vi "PERFORMANCE FUNCTIONS.vi"(0 "Source Name":string="Source Name", 11 "Error In Cluster":T1={"Unhandled Error"=FALSE, "Error"={"status"=FALSE, "code"=0, "source"=""}, "Message Type"=enum."Code", "Number of Values"=0, "Msg Value Type"=[], "Msg Ints"=[], "Msg Real Values"=[], "Msg String Values"=[], "Severity (Emergency)"=enum."Emergency"} {"Msg Real Values" format="%.2f"}) -> (15 "Error Out Cluster":T2={"Unhandled Error"=FALSE, "Error"={"status"=FALSE, "code"=0, "source"=""}, "Message Type"=enum."Code", "Number of Values"=0, "Msg Value Type"=[], "Msg Ints"=[], "Msg Real Values"=[], "Msg String Values"=[], "Severity (Emergency)"=enum."Emergency"} {"Msg Real Values" format="%.2f"})   [LabVIEW 2013, in "Customer.TestSLATE.Mnemonic.lvlib"]
doc: "XXX PERFORMANCE FUNCTIONS.vi monitors the current command set active for the data manager running under the DTMGR EXEC and performs each command as it is received. Valid commands are INIT (Initialize system), ACQ (Data Acquisition), DIAG (Diagnostics), STOP (No command active, but data collection will be performed), CAL\n(Calibration), and RELOAD DB (Collect new required configuration database files)."
uses:
  Customer.TestSLATE.Mnemonic.lvlib
  <vilib>/Test SLATE/CONTROLS/Error Out Cluster.ctl
  <vilib>/Test SLATE/CONTROLS/Error In Cluster.ctl
  <vilib>/Test SLATE/Test SLATE.lvlib
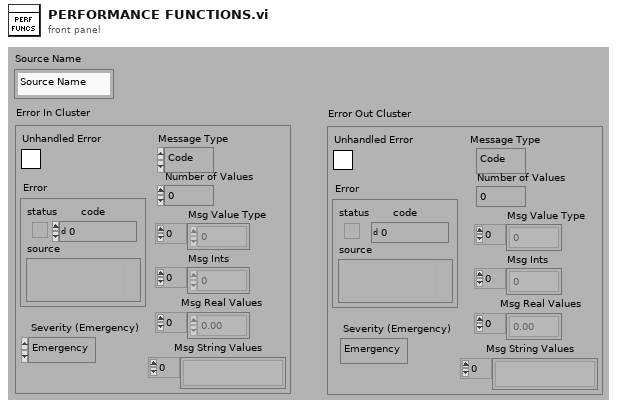
[diagram p1: front panel]
types:
  T1 = typedef "Test SLATE.lvlib/Error In Cluster.ctl" = cluster{"Unhandled Error":bool, "Error":errorcluster, "Message Type":enum8{"Code", "Text"}, "Number of Values":i8, "Msg Value Type":i32[], "Msg Ints":i32[], "Msg Real Values":sgl[], "Msg String Values":string[], "Severity (Emergency)":enum32{"Information", "Warning", "Emergency"}}
  T2 = typedef "Test SLATE.lvlib/Error Out Cluster.ctl" = cluster{"Unhandled Error":bool, "Error":errorcluster, "Message Type":enum8{"Code", "Text"}, "Number of Values":i8, "Msg Value Type":i32[], "Msg Ints":i32[], "Msg Real Values":sgl[], "Msg String Values":string[], "Severity (Emergency)":enum32{"Information", "Warning", "Emergency"}}
  T3 = typedef "Test SLATE.lvlib/Tag Information.ctl" = refnum<class "TS_Tag.lvclass">
  T4 = typedef "Test SLATE.lvlib/CALIBRATION TYPE EXEC.ctl" = enum16{"End to End", "Special 1", "Special 2", "Special 3", "Waiting for Type", "Special 4", "Special 5"}
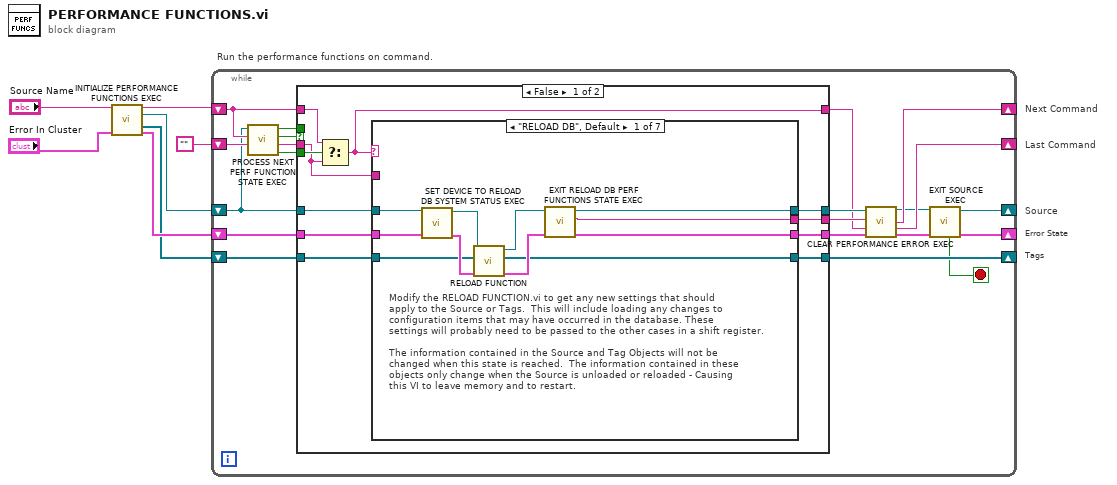
[diagram p0: block diagram]
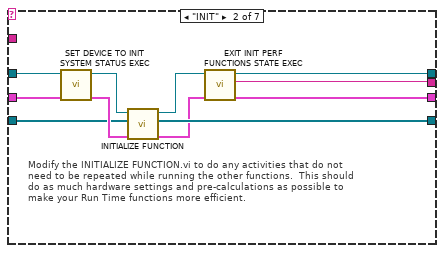
[diagram p2: hidden frame]
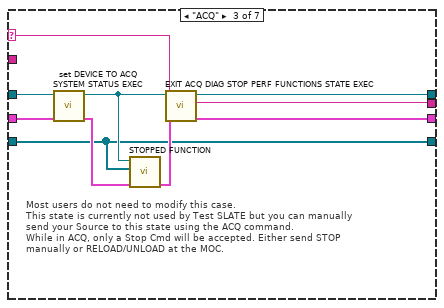
[diagram p3: hidden frame]
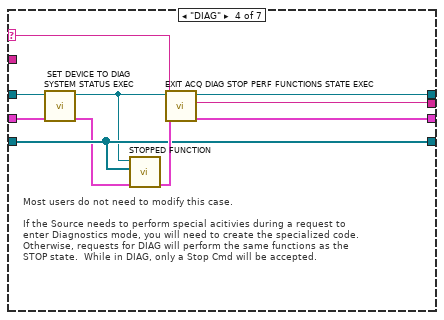
[diagram p4: hidden frame]
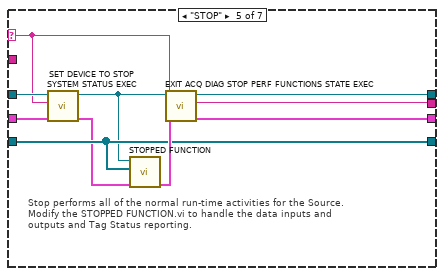
[diagram p5: hidden frame]
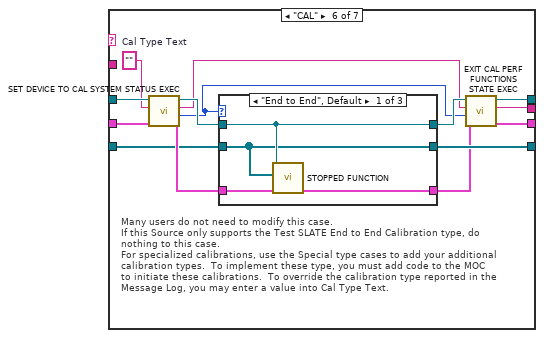
[diagram p6: hidden frame]
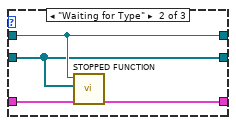
[diagram p7: hidden frame]
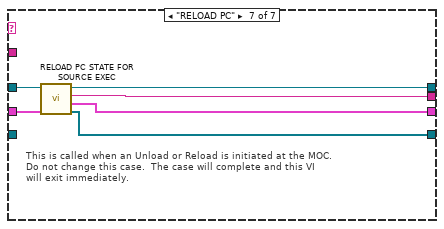
[diagram p9: hidden frame]
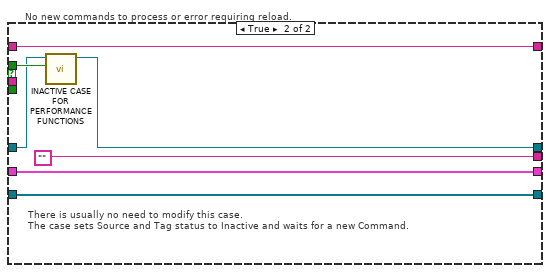
[diagram p10: hidden frame]
diagram:
  # "Tags"
  # "Error State"
  # "Source"
  # "Last Command"
  # "Next Command"
  # "Run the performance functions on command."
  n1 = call <vilib>:"INITIALIZE PERFORMANCE FUNCTIONS EXEC.vi"("Source Name"="Source Name", "Error In Cluster"="Error In Cluster") -> ("Init Command"=w5:string, "Source"=w2:refnum<class "Source.lvclass">, "Tags"=w1:T3[], "Error Out Cluster"=w7:T1)  [unwired: 9 in, 1 out]
  n2 = while {
    shift-left: w5 -> [w19]
    shift-right: [w16] -> _
    shift-left: "" -> [w28]
    shift-right: [w13] -> _
    shift-left: w7 -> [w27]
    shift-right: [w9] -> _
    shift-right: [w21] -> _
    shift-left: w1 -> [w20]
    shift-right: [w11] -> _
    shift-left: w2 -> [w18]
    stop <- w8 stop-if-true
    n3 = call <vilib>:"PROCESS NEXT PERF FUNCTION STATE EXEC.vi"("Last Command"=w28, "Next Command From DTMGR"=w19, "Source"=w18) -> ("Use DTMGR Cmd?"=w26:bool, "Current Command"=w22:string, "Go INACTIVE?"=w25:bool, "MOC sent INACTIVE CMD?"=w23:bool)  [unwired: 5 in]
    n4 = case shown="False" w25 {
      tunnel: [w33 w129] -> w24
      tunnel: w27 -> [w38 w129]
      tunnel: w22 -> [w35 _]
      tunnel: w19 -> [w36 w126]
      tunnel: [w39 w123] -> w15
      tunnel: w26 -> [w37 _]
      tunnel: [w34 w126] -> w14
      tunnel: w23 -> [_ w128]
      tunnel: w18 -> [w32 w124]
      tunnel: [w31 w127] -> w21
      tunnel: w20 -> [w30 w127]
      tunnel: [w29 ""] -> w17
      frame False {
        n5 = Select(t=w36, s=w37, f=w35) -> (s? t:f=w34:string)
        n6 = case shown="\"RELOAD DB\", Default" w34 {
          selector: w34 -> [_ _ w68 w81 w85 _ _]
          tunnel: [w44 w58 w65 w79 w90 w96 w120] -> w33
          tunnel: [w43 w61 w64 w78 w89 w98 w118] -> w39
          tunnel: w38 -> [w50 w59 w71 w75 w86 w105 w121]
          tunnel: w35 -> [_ _ _ _ _ _ _]
          tunnel: w32 -> [w49 w60 w70 w76 w87 w104 w122]
          tunnel: [w45 w55 w63 w77 w88 w100 w119] -> w31
          tunnel: w30 -> [w40 w52 w63 w77 w88 w101 _]
          tunnel: [w41 w51 w62 w72 w82 w95 w117] -> w29
          frame "RELOAD DB", Default {
            # "Modify the RELOAD FUNCTION.vi to get any new settings that should\napply to the Source or Tags.  This will include loading any changes to\nconfiguration items that may have occurred in the database. These \nsettings will probably need to be passed to the other cases in a shift register.\n\nThe information contained in the Source and Tag Objects will not be\nchanged when this state is reached.  The information contained in these\nobjects only change when the Source is unloaded or reloaded - Causing\nthis VI to leave memory and to restart."
            n7 = call <vilib>:"SET DEVICE TO RELOAD DB SYSTEM STATUS EXEC.vi"("Error In Cluster"=w50, "Source"=w49) -> ("Error Out Cluster"=w47:T2, "Source out"=w48:refnum<class "Source.lvclass">)  [unwired: 8 in]
            n8 = call "RELOAD FUNCTION.vi"("Error In Cluster"=w47, "Tags"=w40, "Source"=w48) -> ("Error Out Cluster"=w46:T2, "Tags Out"=w45:T3[], "Source out"=w42:refnum<class "Source.lvclass">)  [unwired: 6 in]
            n9 = call <vilib>:"EXIT RELOAD DB PERF FUNCTIONS STATE EXEC.vi"("Error In Cluster"=w46, "Source"=w42) -> ("Error Out Cluster"=w44:T2, "Next Command"=w41:string, "Source Out"=w43:refnum<class "Source.lvclass">)  [unwired: 7 in]
          }
          frame "INIT" {
            # "Modify the INITIALIZE FUNCTION.vi to do any activities that do not \nneed to be repeated while running the other functions.  This should\ndo as much hardware settings and pre-calculations as possible to\nmake your Run Time functions more efficient."
            n10 = call <vilib>:"SET DEVICE TO INIT SYSTEM STATUS EXEC.vi"("Error In Cluster"=w59, "Source"=w60) -> ("Error Out Cluster"=w54:T1, "Source out"=w57:refnum<class "Source.lvclass">)  [unwired: 6 in]
            n11 = call "INITIALIZE FUNCTION.vi"("Error In Cluster"=w54, "Tags"=w52, "Source"=w57) -> ("Error Out Cluster"=w53:T2, "Tags out"=w55:T3[], "Source out"=w56:refnum<class "Source.lvclass">)  [unwired: 6 in]
            n12 = call <vilib>:"EXIT INIT PERF FUNCTIONS STATE EXEC.vi"("Error In Cluster"=w53, "Source"=w56) -> ("Error Out Cluster"=w58:T1, "Next Command Step"=w51:string, "Source out"=w61:refnum<class "Source.lvclass">)  [unwired: 5 in]
          }
          frame "ACQ" {
            # "Most users do not need to modify this case.\nThis state is currently not used by Test SLATE but you can manually\nsend your Source to this state using the ACQ command.  \nWhile in ACQ, only a Stop Cmd will be accepted. Either send STOP\nmanually or RELOAD/UNLOAD at the MOC."
            n13 = call <vilib>:"set DEVICE TO ACQ SYSTEM STATUS EXEC.vi"("Error In"=w71, "Source"=w70) -> ("Error Out Cluster"=w69:T2, "Source out"=w66:refnum<class "Source.lvclass">)  [unwired: 8 in]
            n14 = call "STOPPED FUNCTION.vi"("Error In Cluster"=w69, "Tags"=w63, "Source"=w66) -> ("Error Out Cluster"=w67:T2)  [unwired: 8 in]
            n15 = call <vilib>:"EXIT ACQ DIAG STOP PERF FUNCTIONS STATE EXEC.vi"("Error In Cluster"=w67, "Command"=w68, "Source"=w66) -> ("Error Out Cluster"=w65:T2, "Next Command"=w62:string, "Source Out"=w64:refnum<class "Source.lvclass">)  [unwired: 6 in]
          }
          frame "DIAG" {
            # "Most users do not need to modify this case.\n\nIf the Source needs to perform special acitivies during a request to\nenter Diagnostics mode, you will need to create the specialized code.\nOtherwise, requests for DIAG will perform the same functions as the \nSTOP state.  While in DIAG, only a Stop Cmd will be accepted."
            n16 = call <vilib>:"SET DEVICE TO DIAG SYSTEM STATUS EXEC.vi"("Error In Cluster"=w75, "Source"=w76) -> ("Error Out Cluster"=w74:T2, "Source out"=w73:refnum<class "Source.lvclass">)  [unwired: 8 in]
            n17 = call "STOPPED FUNCTION.vi"("Error In Cluster"=w74, "Tags"=w77, "Source"=w73) -> ("Error Out Cluster"=w80:T2)  [unwired: 8 in]
            n18 = call <vilib>:"EXIT ACQ DIAG STOP PERF FUNCTIONS STATE EXEC.vi"("Error In Cluster"=w80, "Command"=w81, "Source"=w73) -> ("Error Out Cluster"=w79:T2, "Next Command"=w72:string, "Source Out"=w78:refnum<class "Source.lvclass">)  [unwired: 6 in]
          }
          frame "STOP" {
            # "Stop performs all of the normal run-time activities for the Source.\nModify the STOPPED FUNCTION.vi to handle the data inputs and\noutputs and Tag Status reporting."
            n19 = call <vilib>:"SET DEVICE TO STOP SYSTEM STATUS EXEC.vi"("Error In Cluster"=w86, "MOC Command"=w85, "Source"=w87) -> ("Error Out Cluster"=w83:T2, "Source out"=w84:refnum<class "Source.lvclass">)  [unwired: 6 in]
            n20 = call "STOPPED FUNCTION.vi"("Error In Cluster"=w83, "Tags"=w88, "Source"=w84) -> ("Error Out Cluster"=w91:T2)  [unwired: 8 in]
            n21 = call <vilib>:"EXIT ACQ DIAG STOP PERF FUNCTIONS STATE EXEC.vi"("Error In Cluster"=w91, "Command"=w85, "Source"=w84) -> ("Error Out Cluster"=w90:T2, "Next Command"=w82:string, "Source Out"=w89:refnum<class "Source.lvclass">)  [unwired: 6 in]
          }
          frame "CAL" {
            w92 = ""  # Cal Type Text
            # "Many users do not need to modify this case.\nIf this Source only supports the Test SLATE End to End Calibration type, do\nnothing to this case.\nFor specialized calibrations, use the Special type cases to add your additional\ncalibration types.  To implement these type, you must add code to the MOC\nto initiate these calibrations.  To override the calibration type reported in the\nMessage Log, you may enter a value into Cal Type Text."
            n22 = call <vilib>:"SET DEVICE TO CAL SYSTEM STATUS EXEC.vi"("Error In Cluster"=w105, "Cal Type Text"=w92, "Source"=w104) -> ("Error Out Cluster"=w103:T2, "Calibration Type"=w93:T4, "Cal Type Text Out"=w94:string, "Source out"=w102:refnum<class "Source.lvclass">)  [unwired: 4 in]
            n23 = case shown="\"End to End\", Default" w93 {
              tunnel: w103 -> [w109 w113 w115]
              tunnel: [w108 w112 w115] -> w97
              tunnel: w102 -> [w107 w111 w116]
              tunnel: w101 -> [w106 w110 w114]
              tunnel: [w107 w111 w116] -> w99
              tunnel: [w106 w110 w114] -> w100
              frame "End to End", Default {
                n24 = call "STOPPED FUNCTION.vi"("Error In Cluster"=w109, "Tags"=w106, "Source"=w107) -> ("Error Out Cluster"=w108:T2)  [unwired: 8 in]
              }
              frame "Waiting for Type" {
                # "Put the waiting code here.  \nUsually the same \nas stopped (idle mode)."
                n25 = call "STOPPED FUNCTION.vi"("Error In Cluster"=w113, "Tags"=w110, "Source"=w111) -> ("Error Out Cluster"=w112:T2)  [unwired: 8 in]
              }
              frame "Special 1".."Special 3" {
                # "Add whatever you need for\nthese calibrations.  Use Stop\nAvailable to tell the cmd interface\nif stop commands are available."
              }
            }
            n26 = call <vilib>:"EXIT CAL PERF FUNCTIONS STATE EXEC.vi"("Error In Cluster"=w97, "Calibration Type"=w93, "Cal Type String"=w94, "Source"=w99) -> ("Error Out Cluster"=w96:T2, "Next Command"=w95:string, "Source Out"=w98:refnum<class "Source.lvclass">)  [unwired: 5 in]
          }
          frame "RELOAD PC" {
            # "This is called when an Unload or Reload is initiated at the MOC.\nDo not change this case.  The case will complete and this VI\nwill exit immediately."
            n27 = call <vilib>:"RELOAD PC STATE FOR SOURCE EXEC.vi"("Error In Cluster"=w121, "Source"=w122) -> ("Tags"=w119:T3[], "Error Out Cluster"=w120:T2, "Next Command"=w117:string, "Source Out"=w118:refnum<class "Source.lvclass">)  [unwired: 6 in]
          }
        }
        "Error Out Cluster" <- w33
      }
      frame True {
        # "There is usually no need to modify this case.\nThe case sets Source and Tag status to Inactive and waits for a new Command."
        # "No new commands to process or error requiring reload."
        n28 = call <vilib>:"INACTIVE CASE FOR PERFORMANCE FUNCTIONS.vi"("Stop Status Update Value"=w128, "Source"=w124) -> ("Source Out"=w123:refnum<class "Source.lvclass">)  [unwired: 9 in]
      }
    }
    n29 = call <vilib>:"CLEAR PERFORMANCE ERROR EXEC.vi"("Source"=w15, "Next Command in"=w17, "Last Command in"=w14, "Error In Cluster"=w24) -> ("Source out"=w12:refnum<class "Source.lvclass">, "Next Command Out"=w16:string, "Last Command out"=w13:string, "Error Out Cluster"=w10:T2)  [unwired: 8 in]
    n30 = call <vilib>:"EXIT SOURCE EXEC.vi"("Error In Cluster"=w10, "Source in"=w12) -> ("Error Out Cluster"=w9:T2, "Source out"=w11:refnum<class "Source.lvclass">, "Exit Source?"=w8:bool)  [unwired: 7 in]
  }
